vi "ConnectionHelperVMXTitan.vi"(5 "InCluster":cluster{"Motors":dbl[], "HCDIOValues":dbl[]}, 6 "ErrorIn":errorcluster, 9 "Reference":T1) -> (0 "ErrorOut":errorcluster, 3 "OutReference":T1, 4 "OutCluster":T3)   [LabVIEW 2019]
uses:
  <vilib>/vision/Image Controls.llb/IMAQ Image.ctl
  C:/Users/yasav/Downloads/prev_robocad/robocadSimLVFolder/assemblies/LibraryForLabVIEW.dll
  assemblies/LibraryForLabVIEW.dll
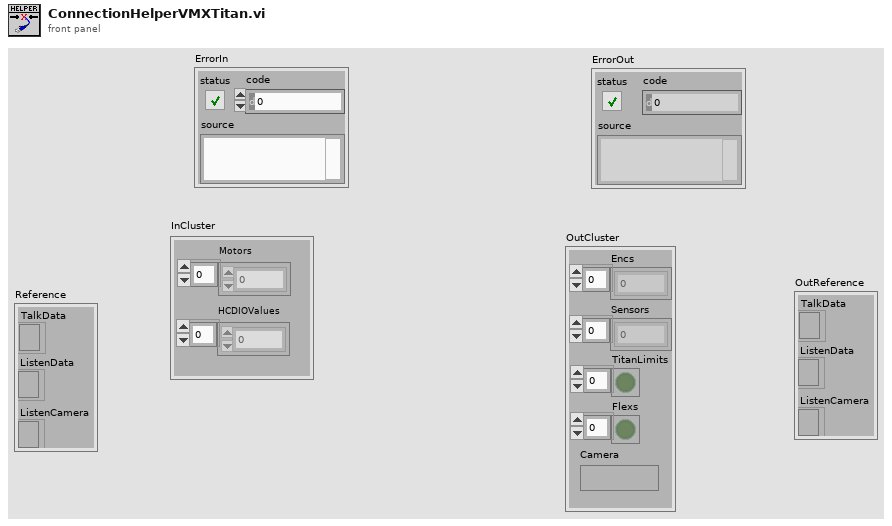
[diagram p1: front panel]
types:
  T1 = cluster{"ListenData":refnum<k24>, "ListenCamera":refnum<k24>, "TalkData":refnum<k24>}
  T2 = typedef "IMAQ Image.ctl" = refnum<image>
  T3 = cluster{"Encs":dbl[], "Sensors":dbl[], "TitanLimits":bool[], "Flexs":bool[], "Camera":T2}
  T4 = typedef "Image Type" = u32
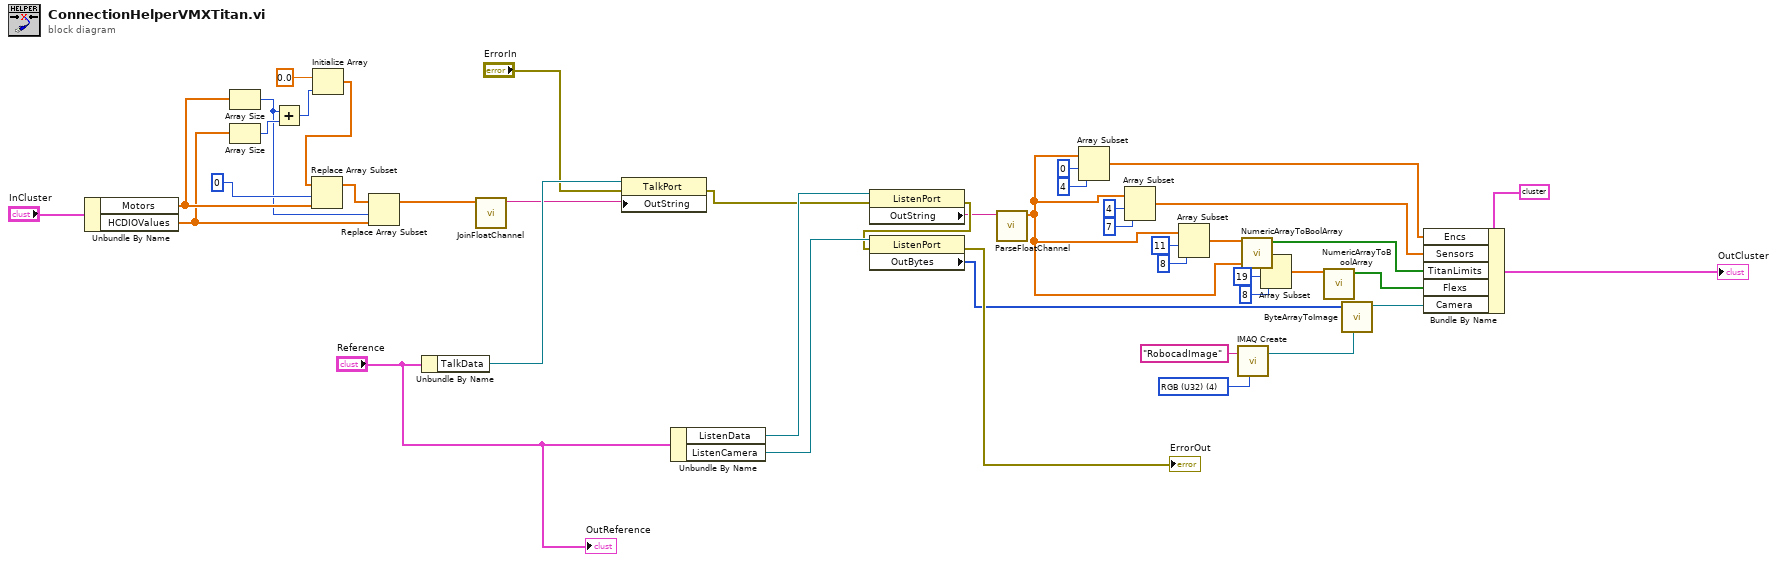
[diagram p0: block diagram]
diagram:
  w20 = T4 4 items=["Grayscale (U8)", "Grayscale (I16)", "Grayscale (SGL)", "Complex (CSG)", "RGB (U32)", "HSL (U32)", "RGB (U64)", "Grayscale (U16)"] ("Image Type")
  n1 = Unbundle By Name("InCluster") -> ("Motors"=w30:dbl[], "HCDIOValues"=w27:dbl[])
  n2 = Array Size(array=w30) -> (size(s)=w26:i32)
  n3 = Array Size(array=w27) -> (size(s)=w33:i32)
  n4 = Add(x=w26, y=w33) -> (x+y=w32:i32)
  n5 = Initialize Array(0.0 ("element"), w32) -> (w31:dbl[])
  n6 = Replace Array Subset(array=w31, new element=w30, index=0) -> (w28:dbl[])
  n7 = Replace Array Subset(array=w28, new element=w27, index=w26) -> (w25:dbl[])
  n8 = Unbundle By Name("Reference") -> ("TalkData"=w42:refnum<k24>)
  n9 = call "JoinFloatChannel.vi"("Array"=w25) -> ("String"=w1:string)  [unwired: 10 in]
  n10 = property class="TalkPort"(reference=w42, error in="ErrorIn", "OutString"=w1) -> (error out=w35:errorcluster)  [unwired: 1 out]
  n11 = Unbundle By Name("Reference") -> ("ListenData"=w40:refnum<k24>, "ListenCamera"=w37:refnum<k24>)
  n12 = property class="ListenPort"(reference=w40, error in=w35) -> (error out=w36:errorcluster, "OutString"=w17:string)  [unwired: 1 out]
  n13 = property class="ListenPort"(reference=w37, error in=w36) -> (error out=→"ErrorOut":errorcluster, "OutBytes"=w21:u8[])  [unwired: 1 out]
  n14 = call "ParseFloatChannel.vi"("Input"=w17) -> ("Array"=w2:dbl[])  [unwired: 10 in]
  n15 = Array Subset(array=w2, index=0, length=4) -> (w14:dbl[])
  n16 = Array Subset(array=w2, index=4, length=7) -> (w11:dbl[])
  n17 = Array Subset(array=w2, index=11, length=8) -> (w8:dbl[])
  n18 = call "IMAQ Create"("Image Name"="RobocadImage", "Image Type"=w20) -> ("New Image"=w18:T2)  [unwired: 3 in, 1 out]
  n19 = call "NumericArrayToBoolArray.vi"("InArray"=w8) -> ("OutArray"=w7:bool[])  [unwired: 10 in]
  n20 = Array Subset(array=w2, index=19, length=8) -> (w4:dbl[])
  n21 = call "NumericArrayToBoolArray.vi"("InArray"=w4) -> ("OutArray"=w3:bool[])  [unwired: 10 in]
  n22 = call "ByteArrayToImage.vi"("CameraBytes"=w21, "Image"=w18) -> ("Image Out"=w22:T2)  [unwired: 6 in]
  n23 = Bundle By Name(cluster=T3 {"Encs"=[], "Sensors"=[], "TitanLimits"=[], "Flexs"=[], "Camera"=refnum} ("OutCluster"), "Encs"=w14, "Sensors"=w11, "TitanLimits"=w7, "Flexs"=w3, "Camera"=w22) -> (→"OutCluster":T3)
  "OutReference" <- "Reference"
